vi "Fetch Measurement (Statistics).vi"(8 "error in (no error)":errorcluster, 10 "Timeout (10000 ms)":u32=10000, 11 "VISA resource name":refnum<visa-resource-name>) -> (0 "error out":errorcluster, 1 "Standard Deviation":dbl, 2 "Mean":dbl format="%#_12g", 3 "VISA resource name out":refnum<visa-resource-name>, 4 "Maximum":dbl format="%#_12g", 5 "Minimum":dbl format="%#_12g")   [LabVIEW 2024, in "Agilent 532XX Series.lvlib"]
doc: "Queries and retrieves measurement statistics.\n\n<B>Note:</B> This VI does not check the instrument status. Typically, you call this VI only in a sequence of calls to other low-level instrument driver VIs. The sequence performs one operation. You use the low-level VIs to optimize one or more aspects of interaction with the instrument."
uses:
  Agilent 532XX Series.lvlib
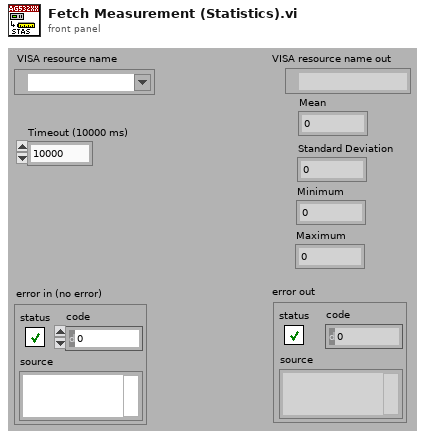
[diagram p1: front panel]
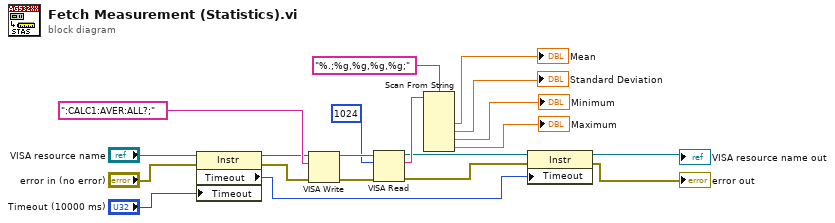
[diagram p0: block diagram]
diagram:
  n1 = property on="Property Node" class="Instr"(reference="VISA resource name", error in="error in (no error)", "Timeout"="Timeout (10000 ms)") -> (reference out=w9:refnum<visa-resource-name>, error out=w8:errorcluster, "Timeout"=w1:u32)
  n2 = VISA Write(VISA resource name=w9, write buffer=":CALC1:AVER:ALL?;", error in (no error)=w8) -> (VISA resource name out=w19:refnum<visa-resource-name>, error out=w18:errorcluster)  [unwired: 1 out]
  n3 = VISA Read(VISA resource name=w19, byte count=u32 1024, error in (no error)=w18) -> (VISA resource name out=w5:refnum<visa-resource-name>, read buffer=w16:string, error out=w2:errorcluster)  [unwired: 1 out]
  n4 = Scan From String(format string="%.;%g,%g,%g,%g;", input string=w16) -> (output 1=→"Mean":dbl, output 2=→"Standard Deviation":dbl, output 3=→"Minimum":dbl, output 4=→"Maximum":dbl)  [unwired: 2 in, 7 out]
  n5 = property on="Property Node" class="Instr"(reference=w5, error in=w2, "Timeout"=w1) -> (reference out=→"VISA resource name out":refnum<visa-resource-name>, error out=→"error out":errorcluster)
